vi "passTestBallOut.vi"(10 "IA state":T2) -> (1 "Result":T1)   [LabVIEW 2017]
uses:
  <extravilib>/ChannelInstances/Lossy Stream-t'AI Input.ctl'/)Channel.ctl
  Core/AI Input.ctl
  Core/AI Robot.ctl
  Intel/Functions Enum.ctl
  Intel/AttackerStates.ctl
  Core/AI Ball.ctl
  Core/Field Size.ctl
  Core/AI Judge.ctl
  Intel/Command Enum.ctl
  Util/Events/Events.ctl
  <extravilib>/ChannelInstances/Lossy Stream-t'passTestStates.ctl'/)Channel.ctl
  passTestStates.ctl
  <extravilib>/ChannelInstances/Lossy Stream-t'AI Input.ctl'/Read With Abort.vi
  <extravilib>/ChannelInstances/Lossy Stream-t'passTestStates.ctl'/Write With Abort.vi
  <extravilib>/ChannelInstances/Lossy Stream-t'AI Input.ctl'/EndpointRead.vi
  <extravilib>/ChannelInstances/Lossy Stream-t'passTestStates.ctl'/Endpoint.vi
  <extravilib>/ChannelInstances/Lossy Stream-t'AI Input.ctl'/)Channel.vi
  <resource>/ChannelSupport/_ChannelSupport/WaitIfNeeded.vi
  <extravilib>/ChannelInstances/Lossy Stream-t'passTestStates.ctl'/)Channel.vi
  <extravilib>/ChannelInstances/Lossy Stream-t'passTestStates.ctl'.lvlib
  <extravilib>/ChannelInstances/Lossy Stream-t'AI Input.ctl'.lvlib
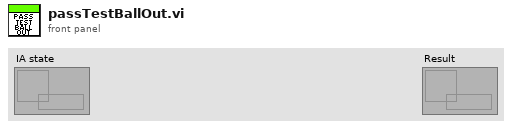
[diagram p1: front panel]
types:
  T1 = typedef "Lossy Stream-t'passTestStates.ctl'.lvlib/)Channel.ctl" = refnum<queue>
  T2 = typedef "Lossy Stream-t'AI Input.ctl'.lvlib/)Channel.ctl" = refnum<queue>
  T3 = typedef "passTestStates.ctl" = enum16{"Pass on the way", "Ball stops", "Pass intercepted", "Ball out of the field", "Ball missed robot", "Need more force to pass", "Too much force", "Correct pass", "Keep ball possesion", "Robot kicked the ball", "Waiting Kick", "Invalid: same robot", "Invalid: kicker ID 999", "Invalid: Receiver ID 999", "Invalid"}
  T4 = typedef "AI Input.ctl" = cluster{"our_robots":T5[], "enemy_robots":T5[], "balls":T8[], "geometry":T9, "IA Judge":T10, "Received Timestamp":timestamp, "Events":T12}
  T5 = typedef "AI Robot.ctl" = cluster{"id":u32, "function":T6, "x":dbl, "y":dbl, "orientation":dbl, "v_tangent":dbl, "v_normal":dbl, "v_ang":dbl, "kick_x":dbl, "kick_z":dbl, "dribble":bool, "Timestamp":timestamp, "dest_x":dbl, "dest_y":dbl, "dest_orientation":dbl, "estimatives":cluster{"est_v_tangent":dbl, "est_v_normal":dbl, "est_vx":dbl, "est_vy":dbl, "Pos Robot Est":dbl[]}, "dest_x_kick":dbl, "dest_y_kick":dbl, "Gap Coord":dbl[], "States":T7}
  T6 = typedef "Functions Enum.ctl" = enum16{"Attacker", "Goalie", "Defender", "Striker", "Goto 0", "Dummy", "Kicker", "ZigZag"}
  T7 = typedef "AttackerStates.ctl" = enum16{"Pass", "GoToTangent", "BallGetting", "GoToKick", ""}
  T8 = typedef "AI Ball.ctl" = cluster{"x":dbl, "y":dbl, "timestamp":timestamp, "Vel_x":dbl, "Vel_y":dbl, "Pos Bola Est":dbl[]}
  T9 = typedef "Field Size.ctl" = cluster{"line_width":u32, "field_length":u32, "field_width":u32, "boundary_width":u32, "referee_width":u32, "goal_width":u32, "goal_depth":u32, "goal_wall_width":u32, "center_circle_radius":u32, "defense_radius":u32, "defense_stretch":u32, "free_kick_from_defense_dist":u32, "penalty_spot_from_field_line_dist":u32, "penalty_line_from_spot_dist":u32}
  T10 = typedef "AI Judge.ctl" = cluster{"stage":string, "command":string, "our_goalie_id":dbl, "enemy_goalie_id":dbl, "command enum":T11, "Time":enum16{"Azul", "Amarelo"}}
  T11 = typedef "Command Enum.ctl" = enum16{"Halt", "Stop", "Force Start", "PKA Normal Start", "Prepare Kickoff Ally", "PKE Normal Start", "Prepare Kickoff Enemy", "Prepare Penalty Ally", "PPA Normal Start", "Prepare Penalty Enemy", "PPE Normal Start", "Direct Free Enemy", "Direct Free Ally", "Indirect Free Enemy", "Indirect Free Ally", "Timeout Enemy", "Timeout Ally", "Goal Enemy", "Goal Ally", "Ball Placement Enemy", "Ball Placement Ally", "Normal Half Time", "Extra Time Break", "Extra Half Time", "None", "Post Game"}
  T12 = typedef "Events.ctl" = cluster{"Touch":bool, "Ball out":bool, "id touch":dbl, "Ball out of \nVision":bool, "Ball inside \nGoalie area":bool, "Robot not responding":bool, "Robots responding status":dbl[], "Enemy Ball \nPossession":bool, "Pass State":bool, "id end of pass":dbl, "Kick":bool, "Id ini Possession":dbl, "Ball Possesion":bool, "Id Possesion":dbl}
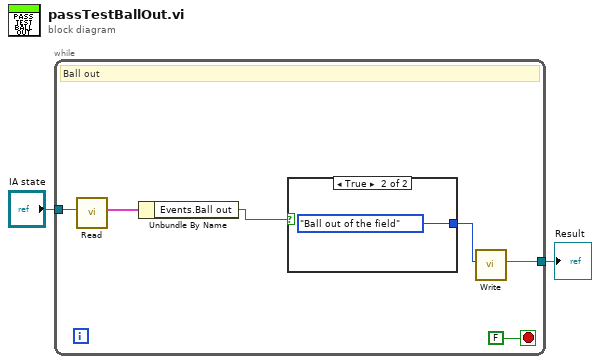
[diagram p0: block diagram]
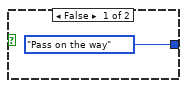
[diagram p2: hidden frame]
diagram:
  n1 = while {
    tunnel: [w7] -> w1
    tunnel: "IA state" -> [w4]
    stop <- FALSE stop-if-true
    # "Ball out"
    n2 = call <extravilib>:"Read.vi"("channel"=w4) -> ("element"=w3:T4)  [unwired: 5 in, 5 out]
    n3 = Unbundle By Name(w3) -> ("Events.Ball out"=w6:bool)
    n4 = case shown="True" w6 {
      tunnel: [passTestStates."Pass on the way" passTestStates."Ball out of the field"] -> w5
      frame False {
      }
      frame True {
      }
    }
    n5 = call <extravilib>:"Write.vi"("element"=w5) -> ("channel"=w7:T1)  [unwired: 8 in, 2 out]
  }
  "Result" <- w1
